vi "Test - Draw Teapot.vi"() -> ()   [LabVIEW 2022 SP3, in "Raster.lvlib"] (continued)
"Vertex 2"={"Position"={"x"=366.29727, "y"=442.02768, "z"=0.9899409}, "UV"={"u"=0.0, "v"=0.0}, "Colour"=12517256}, "Vertex 3"={"Position"={"x"=366.225, "y"=440.50778, "z"=0.990049}, "UV"={"u"=0.0, "v"=0.0}, "Colour"=12517256}, "Alpha"=0.0, "Alpha Blending Enabled"=FALSE, "Colour"=131841}, {"Vertex 1"={"Position"={"x"=433.7027, "y"=442.02768, "z"=0.9899409}, "UV"={"u"=0.0, "v"=0.0}, "Colour"=12517256}, "Vertex 2"={"Position"={"x"=437.2079, "y"=447.81754, "z"=0.98992956}, "UV"={"u"=0.0, "v"=0.0}, "Colour"=12517256}, "Vertex 3"={"Position"={"x"=437.24603, "y"=446.0728, "z"=0.990049}, "UV"={"u"=0.0, "v"=0.0}, "Colour"=12517256}, "Alpha"=0.0, "Alpha Blending Enabled"=FALSE, "Colour"=131841}, {"Vertex 1"={"Position"={"x"=379.34756, "y"=412.01456, "z"=0.98998296}, "UV"={"u"=0.0, "v"=0.0}, "Colour"=12517256}, "Vertex 2"={"Position"={"x"=382.73233, "y"=417.01996, "z"=0.98999375}, "UV"={"u"=0.0, "v"=0.0}, "Colour"=12517256}, "Vertex 3"={"Position"={"x"=383.29828, "y"=417.6338, "z"=0.989941}, "UV"={"u"=0.0, "v"=0.0}, "Colour"=12517256}, "Alpha"=0.0, "Alpha Blending Enabled"=FALSE, "Colour"=6588232}, {"Vertex 1"={"Position"={"x"=382.73233, "y"=417.01996, "z"=0.98999375}, "UV"={"u"=0.0, "v"=0.0}, "Colour"=12517256}, "Vertex 2"={"Position"={"x"=381.5074, "y"=422.85254, "z"=0.98998976}, "UV"={"u"=0.0, "v"=0.0}, "Colour"=12517256}, "Vertex 3"={"Position"={"x"=382.10587, "y"=423.5434, "z"=0.9899332}, "UV"={"u"=0.0, "v"=0.0}, "Colour"=12517256}, "Alpha"=0.0, "Alpha Blending Enabled"=FALSE, "Colour"=197634}, {"Vertex 1"={"Position"={"x"=498.9789, "y"=132.58115, "z"=0.990049}, "UV"={"u"=0.0, "v"=0.0}, "Colour"=12517256}, "Vertex 2"={"Position"={"x"=473.07867, "y"=131.5601, "z"=0.990049}, "UV"={"u"=0.0, "v"=0.0}, "Colour"=12517256}, "Vertex 3"={"Position"={"x"=473.84143, "y"=127.58133, "z"=0.9898128}, "UV"={"u"=0.0, "v"=0.0}, "Colour"=12517256}, "Alpha"=0.0, "Alpha Blending Enabled"=FALSE, "Colour"=131841}, {"Vertex 1"={"Position"={"x"=359.6493, "y"=130.9132, "z"=0.990049}, "UV"={"u"=0.0, "v"=0.0}, "Colour"=12517256}, "Vertex 2"={"Position"={"x"=326.92133, "y"=131.5601, "z"=0.990049}, "UV"={"u"=0.0, "v"=0.0}, "Colour"=12517256}, "Vertex 3"={"Position"={"x"=326.15854, "y"=127.58133, "z"=0.9898128}, "UV"={"u"=0.0, "v"=0.0}, "Colour"=12517256}, "Alpha"=0.0, "Alpha Blending Enabled"=FALSE, "Colour"=131841}, {"Vertex 1"={"Position"={"x"=362.81305, "y"=452.69107, "z"=0.9899296}, "UV"={"u"=0.0, "v"=0.0}, "Colour"=12517256}, "Vertex 2"={"Position"={"x"=362.7921, "y"=447.81754, "z"=0.98992956}, "UV"={"u"=0.0, "v"=0.0}, "Colour"=12517256}, "Vertex 3"={"Position"={"x"=362.754, "y"=446.0728, "z"=0.990049}, "UV"={"u"=0.0, "v"=0.0}, "Colour"=12517256}, "Alpha"=0.0, "Alpha Blending Enabled"=FALSE, "Colour"=724744}, {"Vertex 1"={"Position"={"x"=437.2079, "y"=447.81754, "z"=0.98992956}, "UV"={"u"=0.0, "v"=0.0}, "Colour"=12517256}, "Vertex 2"={"Position"={"x"=437.18695, "y"=452.69107, "z"=0.9899296}, "UV"={"u"=0.0, "v"=0.0}, "Colour"=12517256}, "Vertex 3"={"Position"={"x"=437.22525, "y"=450.8897, "z"=0.990049}, "UV"={"u"=0.0, "v"=0.0}, "Colour"=12517256}, "Alpha"=0.0, "Alpha Blending Enabled"=FALSE, "Colour"=724744}, {"Vertex 1"={"Position"={"x"=758.4817, "y"=387.64502, "z"=0.98992413}, "UV"={"u"=0.0, "v"=0.0}, "Colour"=12517256}, "Vertex 2"={"Position"={"x"=759.2145, "y"=388.6518, "z"=0.9899317}, "UV"={"u"=0.0, "v"=0.0}, "Colour"=12517256}, "Vertex 3"={"Position"={"x"=756.87177, "y"=387.67844, "z"=0.990049}, "UV"={"u"=0.0, "v"=0.0}, "Colour"=12517256}, "Alpha"=0.0, "Alpha Blending Enabled"=FALSE, "Colour"=131841}, {"Vertex 1"={"Position"={"x"=697.0016, "y"=386.77582, "z"=0.9899317}, "UV"={"u"=0.0, "v"=0.0}, "Colour"=12517256}, "Vertex 2"={"Position"={"x"=694.8843, "y"=386.1197, "z"=0.98992413}, "UV"={"u"=0.0, "v"=0.0}, "Colour"=12517256}, "Vertex 3"={"Position"={"x"=689.38416, "y"=385.0128, "z"=0.990049}, "UV"={"u"=0.0, "v"=0.0}, "Colour"=12517256}, "Alpha"=0.0, "Alpha Blending Enabled"=FALSE, "Colour"=9157219}, {"Vertex 1"={"Position"={"x"=422.71338, "y"=429.18945, "z"=0.98997617}, "UV"={"u"=0.0, "v"=0.0}, "Colour"=12517256}, "Vertex 2"={"Position"={"x"=418.4926, "y"=422.85254, "z"=0.98998976}, "UV"={"u"=0.0, "v"=0.0}, "Colour"=12517256}, "Vertex 3"={"Position"={"x"=417.89413, "y"=423.5434, "z"=0.9899332}, "UV"={"u"=0.0, "v"=0.0}, "Colour"=12517256}, "Alpha"=0.0, "Alpha Blending Enabled"=FALSE, "Colour"=131841}, {"Vertex 1"={"Position"={"x"=417.26767, "y"=417.01996, "z"=0.98999375}, "UV"={"u"=0.0, "v"=0.0}, "Colour"=12517256}, "Vertex 2"={"Position"={"x"=420.65244, "y"=412.01456, "z"=0.98998296}, "UV"={"u"=0.0, "v"=0.0}, "Colour"=12517256}, "Vertex 3"={"Position"={"x"=419.99554, "y"=412.71786, "z"=0.9899197}, "UV"={"u"=0.0, "v"=0.0}, "Colour"=12517256}, "Alpha"=0.0, "Alpha Blending Enabled"=FALSE, "Colour"=6653768}, {"Vertex 1"={"Position"={"x"=685.9131, "y"=304.15552, "z"=0.990049}, "UV"={"u"=0.0, "v"=0.0}, "Colour"=12517256}, "Vertex 2"={"Position"={"x"=679.2932, "y"=280.72607, "z"=0.990049}, "UV"={"u"=0.0, "v"=0.0}, "Colour"=12517256}, "Vertex 3"={"Position"={"x"=685.4334, "y"=281.3033, "z"=0.9897971}, "UV"={"u"=0.0, "v"=0.0}, "Colour"=12517256}, "Alpha"=0.0, "Alpha Blending Enabled"=FALSE, "Colour"=131841}, {"Vertex 1"={"Position"={"x"=641.6834, "y"=305.46494, "z"=0.990049}, "UV"={"u"=0.0, "v"=0.0}, "Colour"=12517256}, "Vertex 2"={"Position"={"x"=648.11633, "y"=317.74866, "z"=0.990049}, "UV"={"u"=0.0, "v"=0.0}, "Colour"=12517256}, "Vertex 3"={"Position"={"x"=655.26105, "y"=317.133, "z"=0.9897971}, "UV"={"u"=0.0, "v"=0.0}, "Colour"=12517256}, "Alpha"=0.0, "Alpha Blending Enabled"=FALSE, "Colour"=4941110}, {"Vertex 1"={"Position"={"x"=756.0784, "y"=386.048, "z"=0.9899179}, "UV"={"u"=0.0, "v"=0.0}, "Colour"=12517256}, "Vertex 2"={"Position"={"x"=758.4817, "y"=387.64502, "z"=0.98992413}, "UV"={"u"=0.0, "v"=0.0}, "Colour"=12517256}, "Vertex 3"={"Position"={"x"=755.92346, "y"=386.60867, "z"=0.990049}, "UV"={"u"=0.0, "v"=0.0}, "Colour"=12517256}, "Alpha"=0.0, "Alpha Blending Enabled"=FALSE, "Colour"=131841}, {"Vertex 1"={"Position"={"x"=694.8843, "y"=386.1197, "z"=0.98992413}, "UV"={"u"=0.0, "v"=0.0}, "Colour"=12517256}, "Vertex 2"={"Position"={"x"=692.3103, "y"=384.97452, "z"=0.9899179}, "UV"={"u"=0.0, "v"=0.0}, "Colour"=12517256}, "Vertex 3"={"Position"={"x"=686.6613, "y"=383.84372, "z"=0.990049}, "UV"={"u"=0.0, "v"=0.0}, "Colour"=12517256}, "Alpha"=0.0, "Alpha Blending Enabled"=FALSE, "Colour"=9025634}, {"Vertex 1"={"Position"={"x"=751.9063, "y"=383.8893, "z"=0.9899137}, "UV"={"u"=0.0, "v"=0.0}, "Colour"=12517256}, "Vertex 2"={"Position"={"x"=756.0784, "y"=386.048, "z"=0.9899179}, "UV"={"u"=0.0, "v"=0.0}, "Colour"=12517256}, "Vertex 3"={"Position"={"x"=753.3384, "y"=384.9661, "z"=0.990049}, "UV"={"u"=0.0, "v"=0.0}, "Colour"=12517256}, "Alpha"=0.0, "Alpha Blending Enabled"=FALSE, "Colour"=131841}, {"Vertex 1"={"Position"={"x"=692.3103, "y"=384.97452, "z"=0.9899179}, "UV"={"u"=0.0, "v"=0.0}, "Colour"=12517256}, "Vertex 2"={"Position"={"x"=689.3818, "y"=383.3356, "z"=0.9899137}, "UV"={"u"=0.0, "v"=0.0}, "Colour"=12517256}, "Vertex 3"={"Position"={"x"=683.68915, "y"=382.2069, "z"=0.990049}, "UV"={"u"=0.0, "v"=0.0}, "Colour"=12517256}, "Alpha"=0.0, "Alpha Blending Enabled"=FALSE, "Colour"=8828000}, {"Vertex 1"={"Position"={"x"=745.86945, "y"=381.19867, "z"=0.98991215}, "UV"={"u"=0.0, "v"=0.0}, "Colour"=12517256}, "Vertex 2"={"Position"={"x"=751.9063, "y"=383.8893, "z"=0.9899137}, "UV"={"u"=0.0, "v"=0.0}, "Colour"=12517256}, "Vertex 3"={"Position"={"x"=749.0386, "y"=382.78564, "z"=0.990049}, "UV"={"u"=0.0, "v"=0.0}, "Colour"=12517256}, "Alpha"=0.0, "Alpha Blending Enabled"=FALSE, "Colour"=131841}, {"Vertex 1"={"Position"={"x"=689.3818, "y"=383.3356, "z"=0.9899137}, "UV"={"u"=0.0, "v"=0.0}, "Colour"=12517256}, "Vertex 2"={"Position"={"x"=686.20184, "y"=381.19867, "z"=0.98991215}, "UV"={"u"=0.0, "v"=0.0}, "Colour"=12517256}, "Vertex 3"={"Position"={"x"=680.5922, "y"=380.10245, "z"=0.990049}, "UV"={"u"=0.0, "v"=0.0}, "Colour"=12517256}, "Alpha"=0.0, "Alpha Blending Enabled"=FALSE, "Colour"=8498525}, {"Vertex 1"={"Position"={"x"=381.5074, "y"=422.85254, "z"=0.98998976}, "UV"={"u"=0.0, "v"=0.0}, "Colour"=12517256}, "Vertex 2"={"Position"={"x"=377.28662, "y"=429.18945, "z"=0.98997617}, "UV"={"u"=0.0, "v"=0.0}, "Colour"=12517256}, "Vertex 3"={"Position"={"x"=377.9922, "y"=430.0834, "z"=0.98990643}, "UV"={"u"=0.0, "v"=0.0}, "Colour"=12517256}, "Alpha"=0.0, "Alpha Blending Enabled"=FALSE, "Colour"=131841}, {"Vertex 1"={"Position"={"x"=299.15308, "y"=393.3215, "z"=0.990049}, "UV"={"u"=0.0, "v"=0.0}, "Colour"=12517256}, "Vertex 2"={"Position"={"x"=314.2635, "y"=395.69092, "z"=0.990049}, "UV"={"u"=0.0, "v"=0.0}, "Colour"=12517256}, "Vertex 3"={"Position"={"x"=313.01276, "y"=398.35367, "z"=0.9897707}, "UV"={"u"=0.0, "v"=0.0}, "Colour"=12517256}, "Alpha"=0.0, "Alpha Blending Enabled"=FALSE, "Colour"=8828000}, {"Vertex 1"={"Position"={"x"=470.00256, "y"=398.0604, "z"=0.990049}, "UV"={"u"=0.0, "v"=0.0}, "Colour"=12517256}, "Vertex 2"={"Position"={"x"=485.7365, "y"=395.69092, "z"=0.990049}, "UV"={"u"=0.0, "v"=0.0}, "Colour"=12517256}, "Vertex 3"={"Position"={"x"=486.98724, "y"=398.35367, "z"=0.9897707}, "UV"={"u"=0.0, "v"=0.0}, "Colour"=12517256}, "Alpha"=0.0, "Alpha Blending Enabled"=FALSE, "Colour"=8828000}, {"Vertex 1"={"Position"={"x"=382.10587, "y"=423.5434, "z"=0.9899332}, "UV"={"u"=0.0, "v"=0.0}, "Colour"=12517256}, "Vertex 2"={"Position"={"x"=383.29828, "y"=417.6338, "z"=0.989941}, "UV"={"u"=0.0, "v"=0.0}, "Colour"=12517256}, "Vertex 3"={"Position"={"x"=382.73233, "y"=417.01996, "z"=0.98999375}, "UV"={"u"=0.0, "v"=0.0}, "Colour"=12517256}, "Alpha"=0.0, "Alpha Blending Enabled"=FALSE, "Colour"=197634}, {"Vertex 1"={"Position"={"x"=722.66376, "y"=367.07578, "z"=0.9899058}, "UV"={"u"=0.0, "v"=0.0}, "Colour"=12517256}, "Vertex 2"={"Position"={"x"=745.86945, "y"=381.19867, "z"=0.98991215}, "UV"={"u"=0.0, "v"=0.0}, "Colour"=12517256}, "Vertex 3"={"Position"={"x"=742.9461, "y"=380.10245, "z"=0.990049}, "UV"={"u"=0.0, "v"=0.0}, "Colour"=12517256}, "Alpha"=0.0, "Alpha Blending Enabled"=FALSE, "Colour"=131841}, {"Vertex 1"={"Position"={"x"=686.20184, "y"=381.19867, "z"=0.98991215}, "UV"={"u"=0.0, "v"=0.0}, "Colour"=12517256}, "Vertex 2"={"Position"={"x"=675.37756, "y"=370.58347, "z"=0.9899058}, "UV"={"u"=0.0, "v"=0.0}, "Colour"=12517256}, "Vertex 3"={"Position"={"x"=670.1064, "y"=369.6894, "z"=0.990049}, "UV"={"u"=0.0, "v"=0.0}, "Colour"=12517256}, "Alpha"=0.0, "Alpha Blending Enabled"=FALSE, "Colour"=7576146}, {"Vertex 1"={"Position"={"x"=416.7017, "y"=417.6338, "z"=0.989941}, "UV"={"u"=0.0, "v"=0.0}, "Colour"=12517256}, "Vertex 2"={"Position"={"x"=417.89413, "y"=423.5434, "z"=0.9899332}, "UV"={"u"=0.0, "v"=0.0}, "Colour"=12517256}, "Vertex 3"={"Position"={"x"=418.4926, "y"=422.85254, "z"=0.98998976}, "UV"={"u"=0.0, "v"=0.0}, "Colour"=12517256}, "Alpha"=0.0, "Alpha Blending Enabled"=FALSE, "Colour"=197634}, {"Vertex 1"={"Position"={"x"=679.2932, "y"=280.72607, "z"=0.990049}, "UV"={"u"=0.0, "v"=0.0}, "Colour"=12517256}, "Vertex 2"={"Position"={"x"=671.11444, "y"=257.76425, "z"=0.990049}, "UV"={"u"=0.0, "v"=0.0}, "Colour"=12517256}, "Vertex 3"={"Position"={"x"=678.03265, "y"=257.92834, "z"=0.98976254}, "UV"={"u"=0.0, "v"=0.0}, "Colour"=12517256}, "Alpha"=0.0, "Alpha Blending Enabled"=FALSE, "Colour"=131841}, {"Vertex 1"={"Position"={"x"=632.507, "y"=294.77127, "z"=0.990049}, "UV"={"u"=0.0, "v"=0.0}, "Colour"=12517256}, "Vertex 2"={"Position"={"x"=641.6834, "y"=305.46494, "z"=0.990049}, "UV"={"u"=0.0, "v"=0.0}, "Colour"=12517256}, "Vertex 3"={"Position"={"x"=649.45404, "y"=304.2476, "z"=0.98976254}, "UV"={"u"=0.0, "v"=0.0}, "Colour"=12517256}, "Alpha"=0.0, "Alpha Blending Enabled"=FALSE, "Colour"=6653768}, {"Vertex 1"={"Position"={"x"=371.0727, "y"=408.02982, "z"=0.9899565}, "UV"={"u"=0.0, "v"=0.0}, "Colour"=12517256}, "Vertex 2"={"Position"={"x"=379.34756, "y"=412.01456, "z"=0.98998296}, "UV"={"u"=0.0, "v"=0.0}, "Colour"=12517256}, "Vertex 3"={"Position"={"x"=380.00443, "y"=412.71786, "z"=0.9899197}, "UV"={"u"=0.0, "v"=0.0}, "Colour"=12517256}, "Alpha"=0.0, "Alpha Blending Enabled"=FALSE, "Colour"=8828000}, {"Vertex 1"={"Position"={"x"=419.99554, "y"=412.71786, "z"=0.9899197}, "UV"={"u"=0.0, "v"=0.0}, "Colour"=12517256}, "Vertex 2"={"Position"={"x"=416.7017, "y"=417.6338, "z"=0.989941}, "UV"={"u"=0.0, "v"=0.0}, "Colour"=12517256}, "Vertex 3"={"Position"={"x"=417.26767, "y"=417.01996, "z"=0.98999375}, "UV"={"u"=0.0, "v"=0.0}, "Colour"=12517256}, "Alpha"=0.0, "Alpha Blending Enabled"=FALSE, "Colour"=6588232}, {"Vertex 1"={"Position"={"x"=367.99426, "y"=456.267, "z"=0.98994625}, "UV"={"u"=0.0, "v"=0.0}, "Colour"=12517256}, "Vertex 2"={"Position"={"x"=379.90686, "y"=458.17007, "z"=0.9899845}, "UV"={"u"=0.0, "v"=0.0}, "Colour"=12517256}, "Vertex 3"={"Position"={"x"=380.54544, "y"=459.1382, "z"=0.9899229}, "UV"={"u"=0.0, "v"=0.0}, "Colour"=12517256}, "Alpha"=0.0, "Alpha Blending Enabled"=FALSE, "Colour"=9091427}, {"Vertex 1"={"Position"={"x"=383.29828, "y"=417.6338, "z"=0.989941}, "UV"={"u"=0.0, "v"=0.0}, "Colour"=12517256}, "Vertex 2"={"Position"={"x"=380.00443, "y"=412.71786, "z"=0.9899197}, "UV"={"u"=0.0, "v"=0.0}, "Colour"=12517256}, "Vertex 3"={"Position"={"x"=379.34756, "y"=412.01456, "z"=0.98998296}, "UV"={"u"=0.0, "v"=0.0}, "Colour"=12517256}, "Alpha"=0.0, "Alpha Blending Enabled"=FALSE, "Colour"=6588232}, {"Vertex 1"={"Position"={"x"=707.4174, "y"=348.9724, "z"=0.9898884}, "UV"={"u"=0.0, "v"=0.0}, "Colour"=12517256}, "Vertex 2"={"Position"={"x"=722.66376, "y"=367.07578, "z"=0.9899058}, "UV"={"u"=0.0, "v"=0.0}, "Colour"=12517256}, "Vertex 3"={"Position"={"x"=719.4906, "y"=366.02612, "z"=0.990049}, "UV"={"u"=0.0, "v"=0.0}, "Colour"=12517256}, "Alpha"=0.0, "Alpha Blending Enabled"=FALSE, "Colour"=131841}, {"Vertex 1"={"Position"={"x"=675.37756, "y"=370.58347, "z"=0.9899058}, "UV"={"u"=0.0, "v"=0.0}, "Colour"=12517256}, "Vertex 2"={"Position"={"x"=668.18396, "y"=358.2425, "z"=0.9898884}, "UV"={"u"=0.0, "v"=0.0}, "Colour"=12517256}, "Vertex 3"={"Position"={"x"=662.8006, "y"=357.59274, "z"=0.990049}, "UV"={"u"=0.0, "v"=0.0}, "Colour"=12517256}, "Alpha"=0.0, "Alpha Blending Enabled"=FALSE, "Colour"=5863232}, {"Vertex 1"={"Position"={"x"=359.34708, "y"=404.8941, "z"=0.98991895}, "UV"={"u"=0.0, "v"=0.0}, "Colour"=12517256}, "Vertex 2"={"Position"={"x"=345.11398, "y"=402.38348, "z"=0.9898734}, "UV"={"u"=0.0, "v"=0.0}, "Colour"=12517256}, "Vertex 3"={"Position"={"x"=345.35727, "y"=400.61688, "z"=0.990049}, "UV"={"u"=0.0, "v"=0.0}, "Colour"=12517256}, "Alpha"=0.0, "Alpha Blending Enabled"=FALSE, "Colour"=8827744}, {"Vertex 1"={"Position"={"x"=454.88602, "y"=402.38348, "z"=0.9898734}, "UV"={"u"=0.0, "v"=0.0}, "Colour"=12517256}, "Vertex 2"={"Position"={"x"=440.6529, "y"=404.8941, "z"=0.98991895}, "UV"={"u"=0.0, "v"=0.0}, "Colour"=12517256}, "Vertex 3"={"Position"={"x"=440.6547, "y"=403.54755, "z"=0.990049}, "UV"={"u"=0.0, "v"=0.0}, "Colour"=12517256}, "Alpha"=0.0, "Alpha Blending Enabled"=FALSE, "Colour"=8827744}, {"Vertex 1"={"Position"={"x"=428.32388, "y"=435.69714, "z"=0.9899581}, "UV"={"u"=0.0, "v"=0.0}, "Colour"=12517256}, "Vertex 2"={"Position"={"x"=422.71338, "y"=429.18945, "z"=0.98997617}, "UV"={"u"=0.0, "v"=0.0}, "Colour"=12517256}, "Vertex 3"={"Position"={"x"=422.0078, "y"=430.0834, "z"=0.98990643}, "UV"={"u"=0.0, "v"=0.0}, "Colour"=12517256}, "Alpha"=0.0, "Alpha Blending Enabled"=FALSE, "Colour"=131841}, {"Vertex 1"={"Position"={"x"=400.0, "y"=458.04477, "z"=0.990049}, "UV"={"u"=0.0, "v"=0.0}, "Colour"=12517256}, "Vertex 2"={"Position"={"x"=381.66364, "y"=460.0469, "z"=0.98986506}, "UV"={"u"=0.0, "v"=0.0}, "Colour"=12517256}, "Vertex 3"={"Position"={"x"=380.54544, "y"=459.1382, "z"=0.9899229}, "UV"={"u"=0.0, "v"=0.0}, "Colour"=12517256}, "Alpha"=0.0, "Alpha Blending Enabled"=FALSE, "Colour"=8959842}, {"Vertex 1"={"Position"={"x"=400.0, "y"=458.04477, "z"=0.990049}, "UV"={"u"=0.0, "v"=0.0}, "Colour"=12517256}, "Vertex 2"={"Position"={"x"=419.4546, "y"=459.1382, "z"=0.9899229}, "UV"={"u"=0.0, "v"=0.0}, "Colour"=12517256}, "Vertex 3"={"Position"={"x"=418.33633, "y"=460.0469, "z"=0.98986506}, "UV"={"u"=0.0, "v"=0.0}, "Colour"=12517256}, "Alpha"=0.0, "Alpha Blending Enabled"=FALSE, "Colour"=8959842}, {"Vertex 1"={"Position"={"x"=377.9922, "y"=430.0834, "z"=0.98990643}, "UV"={"u"=0.0, "v"=0.0}, "Colour"=12517256}, "Vertex 2"={"Position"={"x"=382.10587, "y"=423.5434, "z"=0.9899332}, "UV"={"u"=0.0, "v"=0.0}, "Colour"=12517256}, "Vertex 3"={"Position"={"x"=381.5074, "y"=422.85254, "z"=0.98998976}, "UV"={"u"=0.0, "v"=0.0}, "Colour"=12517256}, "Alpha"=0.0, "Alpha Blending Enabled"=FALSE, "Colour"=131841}, {"Vertex 1"={"Position"={"x"=671.11444, "y"=257.76425, "z"=0.990049}, "UV"={"u"=0.0, "v"=0.0}, "Colour"=12517256}, "Vertex 2"={"Position"={"x"=659.06976, "y"=236.3925, "z"=0.990049}, "UV"={"u"=0.0, "v"=0.0}, "Colour"=12517256}, "Vertex 3"={"Position"={"x"=666.5512, "y"=236.05386, "z"=0.9897306}, "UV"={"u"=0.0, "v"=0.0}, "Colour"=12517256}, "Alpha"=0.0, "Alpha Blending Enabled"=FALSE, "Colour"=131841}, {"Vertex 1"={"Position"={"x"=619.40234, "y"=286.3223, "z"=0.990049}, "UV"={"u"=0.0, "v"=0.0}, "Colour"=12517256}, "Vertex 2"={"Position"={"x"=632.507, "y"=294.77127, "z"=0.990049}, "UV"={"u"=0.0, "v"=0.0}, "Colour"=12517256}, "Vertex 3"={"Position"={"x"=640.6776, "y"=292.91815, "z"=0.9897306}, "UV"={"u"=0.0, "v"=0.0}, "Colour"=12517256}, "Alpha"=0.0, "Alpha Blending Enabled"=FALSE, "Colour"=8366683}, {"Vertex 1"={"Position"={"x"=518.84644, "y"=133.92955, "z"=0.990049}, "UV"={"u"=0.0, "v"=0.0}, "Colour"=12517256}, "Vertex 2"={"Position"={"x"=498.9789, "y"=132.58115, "z"=0.990049}, "UV"={"u"=0.0, "v"=0.0}, "Colour"=12517256}, "Vertex 3"={"Position"={"x"=500.85635, "y"=127.179695, "z"=0.98972636}, "UV"={"u"=0.0, "v"=0.0}, "Colour"=12517256}, "Alpha"=0.0, "Alpha Blending Enabled"=FALSE, "Colour"=131841}, {"Vertex 1"={"Position"={"x"=326.92133, "y"=131.5601, "z"=0.990049}, "UV"={"u"=0.0, "v"=0.0}, "Colour"=12517256}, "Vertex 2"={"Position"={"x"=301.0211, "y"=132.58115, "z"=0.990049}, "UV"={"u"=0.0, "v"=0.0}, "Colour"=12517256}, "Vertex 3"={"Position"={"x"=299.14365, "y"=127.179695, "z"=0.98972636}, "UV"={"u"=0.0, "v"=0.0}, "Colour"=12517256}, "Alpha"=0.0, "Alpha Blending Enabled"=FALSE, "Colour"=131841}, {"Vertex 1"={"Position"={"x"=285.66385, "y"=390.76498, "z"=0.990049}, "UV"={"u"=0.0, "v"=0.0}, "Colour"=12517256}, "Vertex 2"={"Position"={"x"=299.15308, "y"=393.3215, "z"=0.990049}, "UV"={"u"=0.0, "v"=0.0}, "Colour"=12517256}, "Vertex 3"={"Position"={"x"=297.17767, "y"=396.39102, "z"=0.98972005}, "UV"={"u"=0.0, "v"=0.0}, "Colour"=12517256}, "Alpha"=0.0, "Alpha Blending Enabled"=FALSE, "Colour"=8828000}, {"Vertex 1"={"Position"={"x"=485.7365, "y"=395.69092, "z"=0.990049}, "UV"={"u"=0.0, "v"=0.0}, "Colour"=12517256}, "Vertex 2"={"Position"={"x"=500.84695, "y"=393.3215, "z"=0.990049}, "UV"={"u"=0.0, "v"=0.0}, "Colour"=12517256}, "Vertex 3"={"Position"={"x"=502.8223, "y"=396.39102, "z"=0.98972005}, "UV"={"u"=0.0, "v"=0.0}, "Colour"=12517256}, "Alpha"=0.0, "Alpha Blending Enabled"=FALSE, "Colour"=8828000}, {"Vertex 1"={"Position"={"x"=176.70644, "y"=203.00851, "z"=0.9898844}, "UV"={"u"=0.0, "v"=0.0}, "Colour"=12517256}, "Vertex 2"={"Position"={"x"=198.99898, "y"=192.16704, "z"=0.9898844}, "UV"={"u"=0.0, "v"=0.0}, "Colour"=12517256}, "Vertex 3"={"Position"={"x"=202.54619, "y"=193.041, "z"=0.990049}, "UV"={"u"=0.0, "v"=0.0}, "Colour"=12517256}, "Alpha"=0.0, "Alpha Blending Enabled"=FALSE, "Colour"=131841}, {"Vertex 1"={"Position"={"x"=189.0271, "y"=222.08267, "z"=0.9898844}, "UV"={"u"=0.0, "v"=0.0}, "Colour"=12517256}, "Vertex 2"={"Position"={"x"=173.90924, "y"=229.9663, "z"=0.9898844}, "UV"={"u"=0.0, "v"=0.0}, "Colour"=12517256}, "Vertex 3"={"Position"={"x"=177.49036, "y"=231.8874, "z"=0.990049}, "UV"={"u"=0.0, "v"=0.0}, "Colour"=12517256}, "Alpha"=0.0, "Alpha Blending Enabled"=FALSE, "Colour"=8498525}, {"Vertex 1"={"Position"={"x"=156.89874, "y"=214.32089, "z"=0.9898844}, "UV"={"u"=0.0, "v"=0.0}, "Colour"=12517256}, "Vertex 2"={"Position"={"x"=176.70644, "y"=203.00851, "z"=0.9898844}, "UV"={"u"=0.0, "v"=0.0}, "Colour"=12517256}, "Vertex 3"={"Position"={"x"=180.40538, "y"=203.79315, "z"=0.990049}, "UV"={"u"=0.0, "v"=0.0}, "Colour"=12517256}, "Alpha"=0.0, "Alpha Blending Enabled"=FALSE, "Colour"=131841}, {"Vertex 1"={"Position"={"x"=173.90924, "y"=229.9663, "z"=0.9898844}, "UV"={"u"=0.0, "v"=0.0}, "Colour"=12517256}, "Vertex 2"={"Position"={"x"=160.64813, "y"=238.9713, "z"=0.9898844}, "UV"={"u"=0.0, "v"=0.0}, "Colour"=12517256}, "Vertex 3"={"Position"={"x"=164.63506, "y"=240.6793, "z"=0.990049}, "UV"={"u"=0.0, "v"=0.0}, "Colour"=12517256}, "Alpha"=0.0, "Alpha Blending Enabled"=FALSE, "Colour"=7971671}, {"Vertex 1"={"Position"={"x"=139.54333, "y"=226.07301, "z"=0.9898844}, "UV"={"u"=0.0, "v"=0.0}, "Colour"=12517256}, "Vertex 2"={"Position"={"x"=156.89874, "y"=214.32089, "z"=0.9898844}, "UV"={"u"=0.0, "v"=0.0}, "Colour"=12517256}, "Vertex 3"={"Position"={"x"=160.72755, "y"=214.98953, "z"=0.990049}, "UV"={"u"=0.0, "v"=0.0}, "Colour"=12517256}, "Alpha"=0.0, "Alpha Blending Enabled"=FALSE, "Colour"=131841}, {"Vertex 1"={"Position"={"x"=160.64813, "y"=238.9713, "z"=0.9898844}, "UV"={"u"=0.0, "v"=0.0}, "Colour"=12517256}, "Vertex 2"={"Position"={"x"=149.1812, "y"=248.82013, "z"=0.9898844}, "UV"={"u"=0.0, "v"=0.0}, "Colour"=12517256}, "Vertex 3"={"Position"={"x"=153.52568, "y"=250.31297, "z"=0.990049}, "UV"={"u"=0.0, "v"=0.0}, "Colour"=12517256}, "Alpha"=0.0, "Alpha Blending Enabled"=FALSE, "Colour"=7444305}, {"Vertex 1"={"Position"={"x"=124.60768, "y"=238.23384, "z"=0.9898844}, "UV"={"u"=0.0, "v"=0.0}, "Colour"=12517256}, "Vertex 2"={"Position"={"x"=139.54333, "y"=226.07301, "z"=0.9898844}, "UV"={"u"=0.0, "v"=0.0}, "Colour"=12517256}, "Vertex 3"={"Position"={"x"=143.48154, "y"=226.60681, "z"=0.990049}, "UV"={"u"=0.0, "v"=0.0}, "Colour"=12517256}, "Alpha"=0.0, "Alpha Blending Enabled"=FALSE, "Colour"=131841}, {"Vertex 1"={"Position"={"x"=149.1812, "y"=248.82013, "z"=0.9898844}, "UV"={"u"=0.0, "v"=0.0}, "Colour"=12517256}, "Vertex 2"={"Position"={"x"=139.44592, "y"=259.23462, "z"=0.9898844}, "UV"={"u"=0.0, "v"=0.0}, "Colour"=12517256}, "Vertex 3"={"Position"={"x"=144.09988, "y"=260.50784, "z"=0.990049}, "UV"={"u"=0.0, "v"=0.0}, "Colour"=12517256}, "Alpha"=0.0, "Alpha Blending Enabled"=FALSE, "Colour"=6785610}, {"Vertex 1"={"Position"={"x"=112.05928, "y"=250.77232, "z"=0.9898844}, "UV"={"u"=0.0, "v"=0.0}, "Colour"=12517256}, "Vertex 2"={"Position"={"x"=124.60768, "y"=238.23384, "z"=0.9898844}, "UV"={"u"=0.0, "v"=0.0}, "Colour"=12517256}, "Vertex 3"={"Position"={"x"=128.63612, "y"=238.62166, "z"=0.990049}, "UV"={"u"=0.0, "v"=0.0}, "Colour"=12517256}, "Alpha"=0.0, "Alpha Blending Enabled"=FALSE, "Colour"=131841}, {"Vertex 1"={"Position"={"x"=139.44592, "y"=259.23462, "z"=0.9898844}, "UV"={"u"=0.0, "v"=0.0}, "Colour"=12517256}, "Vertex 2"={"Position"={"x"=131.37982, "y"=269.93704, "z"=0.9898844}, "UV"={"u"=0.0, "v"=0.0}, "Colour"=12517256}, "Vertex 3"={"Position"={"x"=136.29527, "y"=270.98328, "z"=0.990049}, "UV"={"u"=0.0, "v"=0.0}, "Colour"=12517256}, "Alpha"=0.0, "Alpha Blending Enabled"=FALSE, "Colour"=6126915}, {"Vertex 1"={"Position"={"x"=101.86548, "y"=263.65726, "z"=0.9898844}, "UV"={"u"=0.0, "v"=0.0}, "Colour"=12517256}, "Vertex 2"={"Position"={"x"=112.05928, "y"=250.77232, "z"=0.9898844}, "UV"={"u"=0.0, "v"=0.0}, "Colour"=12517256}, "Vertex 3"={"Position"={"x"=116.16016, "y"=251.01059, "z"=0.990049}, "UV"={"u"=0.0, "v"=0.0}, "Colour"=12517256}, "Alpha"=0.0, "Alpha Blending Enabled"=FALSE, "Colour"=131841}, {"Vertex 1"={"Position"={"x"=131.37982, "y"=269.93704, "z"=0.9898844}, "UV"={"u"=0.0, "v"=0.0}, "Colour"=12517256}, "Vertex 2"={"Position"={"x"=124.920364, "y"=280.6494, "z"=0.9898844}, "UV"={"u"=0.0, "v"=0.0}, "Colour"=12517256}, "Vertex 3"={"Position"={"x"=130.04947, "y"=281.45874, "z"=0.990049}, "UV"={"u"=0.0, "v"=0.0}, "Colour"=12517256}, "Alpha"=0.0, "Alpha Blending Enabled"=FALSE, "Colour"=5402171}, {"Vertex 1"={"Position"={"x"=93.99359, "y"=276.8578, "z"=0.9898844}, "UV"={"u"=0.0, "v"=0.0}, "Colour"=12517256}, "Vertex 2"={"Position"={"x"=101.86548, "y"=263.65726, "z"=0.9898844}, "UV"={"u"=0.0, "v"=0.0}, "Colour"=12517256}, "Vertex 3"={"Position"={"x"=106.02248, "y"=263.75024, "z"=0.990049}, "UV"={"u"=0.0, "v"=0.0}, "Colour"=12517256}, "Alpha"=0.0, "Alpha Blending Enabled"=FALSE, "Colour"=131841}, {"Vertex 1"={"Position"={"x"=124.920364, "y"=280.6494, "z"=0.9898844}, "UV"={"u"=0.0, "v"=0.0}, "Colour"=12517256}, "Vertex 2"={"Position"={"x"=120.0052, "y"=291.09393, "z"=0.9898844}, "UV"={"u"=0.0, "v"=0.0}, "Colour"=12517256}, "Vertex 3"={"Position"={"x"=125.30017, "y"=291.65356, "z"=0.990049}, "UV"={"u"=0.0, "v"=0.0}, "Colour"=12517256}, "Alpha"=0.0, "Alpha Blending Enabled"=FALSE, "Colour"=4677427}, {"Vertex 1"={"Position"={"x"=88.41114, "y"=290.34256, "z"=0.9898844}, "UV"={"u"=0.0, "v"=0.0}, "Colour"=12517256}, "Vertex 2"={"Position"={"x"=93.99359, "y"=276.8578, "z"=0.9898844}, "UV"={"u"=0.0, "v"=0.0}, "Colour"=12517256}, "Vertex 3"={"Position"={"x"=98.19188, "y"=276.81717, "z"=0.990049}, "UV"={"u"=0.0, "v"=0.0}, "Colour"=12517256}, "Alpha"=0.0, "Alpha Blending Enabled"=FALSE, "Colour"=131841}, {"Vertex 1"={"Position"={"x"=120.0052, "y"=291.09393, "z"=0.9898844}, "UV"={"u"=0.0, "v"=0.0}, "Colour"=12517256}, "Vertex 2"={"Position"={"x"=116.571785, "y"=300.99258, "z"=0.9898844}, "UV"={"u"=0.0, "v"=0.0}, "Colour"=12517256}, "Vertex 3"={"Position"={"x"=121.985054, "y"=301.2872, "z"=0.990049}, "UV"={"u"=0.0, "v"=0.0}, "Colour"=12517256}, "Alpha"=0.0, "Alpha Blending Enabled"=FALSE, "Colour"=3820841}, {"Vertex 1"={"Position"={"x"=85.085556, "y"=304.08072, "z"=0.9898844}, "UV"={"u"=0.0, "v"=0.0}, "Colour"=12517256}, "Vertex 2"={"Position"={"x"=88.41114, "y"=290.34256, "z"=0.9898844}, "UV"={"u"=0.0, "v"=0.0}, "Colour"=12517256}, "Vertex 3"={"Position"={"x"=92.63716, "y"=290.18823, "z"=0.990049}, "UV"={"u"=0.0, "v"=0.0}, "Colour"=12517256}, "Alpha"=0.0, "Alpha Blending Enabled"=FALSE, "Colour"=131841}, {"Vertex 1"={"Position"={"x"=116.571785, "y"=300.99258, "z"=0.9898844}, "UV"={"u"=0.0, "v"=0.0}, "Colour"=12517256}, "Vertex 2"={"Position"={"x"=114.557556, "y"=310.0675, "z"=0.9898844}, "UV"={"u"=0.0, "v"=0.0}, "Colour"=12517256}, "Vertex 3"={"Position"={"x"=120.04168, "y"=310.0791, "z"=0.990049}, "UV"={"u"=0.0, "v"=0.0}, "Colour"=12517256}, "Alpha"=0.0, "Alpha Blending Enabled"=FALSE, "Colour"=2832927}, {"Vertex 1"={"Position"={"x"=83.98433, "y"=318.0409, "z"=0.9898844}, "UV"={"u"=0.0, "v"=0.0}, "Colour"=12517256}, "Vertex 2"={"Position"={"x"=85.085556, "y"=304.08072, "z"=0.9898844}, "UV"={"u"=0.0, "v"=0.0}, "Colour"=12517256}, "Vertex 3"={"Position"={"x"=89.32722, "y"=303.83978, "z"=0.990049}, "UV"={"u"=0.0, "v"=0.0}, "Colour"=12517256}, "Alpha"=0.0, "Alpha Blending Enabled"=FALSE, "Colour"=197634}, {"Vertex 1"={"Position"={"x"=114.557556, "y"=310.0675, "z"=0.9898844}, "UV"={"u"=0.0, "v"=0.0}, "Colour"=12517256}, "Vertex 2"={"Position"={"x"=113.89995, "y"=318.0409, "z"=0.9898844}, "UV"={"u"=0.0, "v"=0.0}, "Colour"=12517256}, "Vertex 3"={"Position"={"x"=119.407745, "y"=317.74866, "z"=0.990049}, "UV"={"u"=0.0, "v"=0.0}, "Colour"=12517256}, "Alpha"=0.0, "Alpha Blending Enabled"=FALSE, "Colour"=1646866}, {"Vertex 1"={"Position"={"x"=85.559654, "y"=330.7427, "z"=0.9898844}, "UV"={"u"=0.0, "v"=0.0}, "Colour"=12517256}, "Vertex 2"={"Position"={"x"=83.98433, "y"=318.0409, "z"=0.9898844}, "UV"={"u"=0.0, "v"=0.0}, "Colour"=12517256}, "Vertex 3"={"Position"={"x"=88.23085, "y"=317.74866, "z"=0.990049}, "UV"={"u"=0.0, "v"=0.0}, "Colour"=12517256}, "Alpha"=0.0, "Alpha Blending Enabled"=FALSE, "Colour"=1976598}, {"Vertex 1"={"Position"={"x"=113.89995, "y"=318.0409, "z"=0.9898844}, "UV"={"u"=0.0, "v"=0.0}, "Colour"=12517256}, "Vertex 2"={"Position"={"x"=115.16618, "y"=324.6623, "z"=0.9898844}, "UV"={"u"=0.0, "v"=0.0}, "Colour"=12517256}, "Vertex 3"={"Position"={"x"=120.644424, "y"=324.08536, "z"=0.990049}, "UV"={"u"=0.0, "v"=0.0}, "Colour"=12517256}, "Alpha"=0.0, "Alpha Blending Enabled"=FALSE, "Colour"=131841}, {"Vertex 1"={"Position"={"x"=90.28456, "y"=340.91348, "z"=0.9898844}, "UV"={"u"=0.0, "v"=0.0}, "Colour"=12517256}, "Vertex 2"={"Position"={"x"=85.559654, "y"=330.7427, "z"=0.9898844}, "UV"={"u"=0.0, "v"=0.0}, "Colour"=12517256}, "Vertex 3"={"Position"={"x"=89.7897, "y"=330.4221, "z"=0.990049}, "UV"={"u"=0.0, "v"=0.0}, "Colour"=12517256}, "Alpha"=0.0, "Alpha Blending Enabled"=FALSE, "Colour"=4611634}, {"Vertex 1"={"Position"={"x"=115.16618, "y"=324.6623, "z"=0.9898844}, "UV"={"u"=0.0, "v"=0.0}, "Colour"=12517256}, "Vertex 2"={"Position"={"x"=118.92371, "y"=329.9643, "z"=0.9898844}, "UV"={"u"=0.0, "v"=0.0}, "Colour"=12517256}, "Vertex 3"={"Position"={"x"=124.31293, "y"=329.15936, "z"=0.990049}, "UV"={"u"=0.0, "v"=0.0}, "Colour"=12517256}, "Alpha"=0.0, "Alpha Blending Enabled"=FALSE, "Colour"=131841}, {"Vertex 1"={"Position"={"x"=98.157074, "y"=348.83447, "z"=0.9898844}, "UV"={"u"=0.0, "v"=0.0}, "Colour"=12517256}, "Vertex 2"={"Position"={"x"=90.28456, "y"=340.91348, "z"=0.9898844}, "UV"={"u"=0.0, "v"=0.0}, "Colour"=12517256}, "Vertex 3"={"Position"={"x"=94.46621, "y"=340.57016, "z"=0.990049}, "UV"={"u"=0.0, "v"=0.0}, "Colour"=12517256}, "Alpha"=0.0, "Alpha Blending Enabled"=FALSE, "Colour"=7049293}, {"Vertex 1"={"Position"={"x"=118.92371, "y"=329.9643, "z"=0.9898844}, "UV"={"u"=0.0, "v"=0.0}, "Colour"=12517256}, "Vertex 2"={"Position"={"x"=125.11115, "y"=334.09354, "z"=0.9898844}, "UV"={"u"=0.0, "v"=0.0}, "Colour"=12517256}, "Vertex 3"={"Position"={"x"=130.35083, "y"=333.11105, "z"=0.990049}, "UV"={"u"=0.0, "v"=0.0}, "Colour"=12517256}, "Alpha"=0.0, "Alpha Blending Enabled"=FALSE, "Colour"=131841}, {"Vertex 1"={"Position"={"x"=109.17566, "y"=354.78696, "z"=0.9898844}, "UV"={"u"=0.0, "v"=0.0}, "Colour"=12517256}, "Vertex 2"={"Position"={"x"=98.157074, "y"=348.83447, "z"=0.9898844}, "UV"={"u"=0.0, "v"=0.0}, "Colour"=12517256}, "Vertex 3"={"Position"={"x"=102.260445, "y"=348.47348, "z"=0.990049}, "UV"={"u"=0.0, "v"=0.0}, "Colour"=12517256}, "Alpha"=0.0, "Alpha Blending Enabled"=FALSE, "Colour"=8564317}, {"Vertex 1"={"Position"={"x"=125.11115, "y"=334.09354, "z"=0.9898844}, "UV"={"u"=0.0, "v"=0.0}, "Colour"=12517256}, "Vertex 2"={"Position"={"x"=133.66658, "y"=337.1965, "z"=0.9898844}, "UV"={"u"=0.0, "v"=0.0}, "Colour"=12517256}, "Vertex 3"={"Position"={"x"=138.69586, "y"=336.0807, "z"=0.990049}, "UV"={"u"=0.0, "v"=0.0}, "Colour"=12517256}, "Alpha"=0.0, "Alpha Blending Enabled"=FALSE, "Colour"=131841}, {"Vertex 1"={"Position"={"x"=123.33839, "y"=359.05215, "z"=0.9898844}, "UV"={"u"=0.0, "v"=0.0}, "Colour"=12517256}, "Vertex 2"={"Position"={"x"=109.17566, "y"=354.78696, "z"=0.9898844}, "UV"={"u"=0.0, "v"=0.0}, "Colour"=12517256}, "Vertex 3"={"Position"={"x"=113.172386, "y"=354.4127, "z"=0.990049}, "UV"={"u"=0.0, "v"=0.0}, "Colour"=12517256}, "Alpha"=0.0, "Alpha Blending Enabled"=FALSE, "Colour"=9157476}, {"Vertex 1"={"Position"={"x"=133.66658, "y"=337.1965, "z"=0.9898844}, "UV"={"u"=0.0, "v"=0.0}, "Colour"=12517256}, "Vertex 2"={"Position"={"x"=144.52863, "y"=339.41995, "z"=0.9898844}, "UV"={"u"=0.0, "v"=0.0}, "Colour"=12517256}, "Vertex 3"={"Position"={"x"=149.28564, "y"=338.2085, "z"=0.990049}, "UV"={"u"=0.0, "v"=0.0}, "Colour"=12517256}, "Alpha"=0.0, "Alpha Blending Enabled"=FALSE, "Colour"=131841}, {"Vertex 1"={"Position"={"x"=140.6435, "y"=361.91113, "z"=0.9898844}, "UV"={"u"=0.0, "v"=0.0}, "Colour"=12517256}, "Vertex 2"={"Position"={"x"=123.33839, "y"=359.05215, "z"=0.9898844}, "UV"={"u"=0.0, "v"=0.0}, "Colour"=12517256}, "Vertex 3"={"Position"={"x"=127.20199, "y"=358.6683, "z"=0.990049}, "UV"={"u"=0.0, "v"=0.0}, "Colour"=12517256}, "Alpha"=0.0, "Alpha Blending Enabled"=FALSE, "Colour"=9420902}, {"Vertex 1"={"Position"={"x"=144.52863, "y"=339.41995, "z"=0.9898844}, "UV"={"u"=0.0, "v"=0.0}, "Colour"=12517256}, "Vertex 2"={"Position"={"x"=157.63564, "y"=340.9104, "z"=0.9898844}, "UV"={"u"=0.0, "v"=0.0}, "Colour"=12517256}, "Vertex 3"={"Position"={"x"=162.05779, "y"=339.6349, "z"=0.990049}, "UV"={"u"=0.0, "v"=0.0}, "Colour"=12517256}, "Alpha"=0.0, "Alpha Blending Enabled"=FALSE, "Colour"=131841}, {"Vertex 1"={"Position"={"x"=161.08936, "y"=363.6454, "z"=0.9898844}, "UV"={"u"=0.0, "v"=0.0}, "Colour"=12517256}, "Vertex 2"={"Position"={"x"=140.6435, "y"=361.91113, "z"=0.9898844}, "UV"={"u"=0.0, "v"=0.0}, "Colour"=12517256}, "Vertex 3"={"Position"={"x"=144.34929, "y"=361.5211, "z"=0.990049}, "UV"={"u"=0.0, "v"=0.0}, "Colour"=12517256}, "Alpha"=0.0, "Alpha Blending Enabled"=FALSE, "Colour"=9486695}, {"Vertex 1"={"Position"={"x"=157.63564, "y"=340.9104, "z"=0.9898844}, "UV"={"u"=0.0, "v"=0.0}, "Colour"=12517256}, "Vertex 2"={"Position"={"x"=172.92587, "y"=341.81445, "z"=0.9898844}, "UV"={"u"=0.0, "v"=0.0}, "Colour"=12517256}, "Vertex 3"={"Position"={"x"=176.94994, "y"=340.5, "z"=0.990049}, "UV"={"u"=0.0, "v"=0.0}, "Colour"=12517256}, "Alpha"=0.0, "Alpha Blending Enabled"=FALSE, "Colour"=131841}, {"Vertex 1"={"Position"={"x"=184.6739, "y"=364.53586, "z"=0.9898844}, "UV"={"u"=0.0, "v"=0.0}, "Colour"=12517256}, "Vertex 2"={"Position"={"x"=161.08936, "y"=363.6454, "z"=0.9898844}, "UV"={"u"=0.0, "v"=0.0}, "Colour"=12517256}, "Vertex 3"={"Position"={"x"=164.61427, "y"=363.25134, "z"=0.990049}, "UV"={"u"=0.0, "v"=0.0}, "Colour"=12517256}, "Alpha"=0.0, "Alpha Blending Enabled"=FALSE, "Colour"=9486951}, {"Vertex 1"={"Position"={"x"=172.92587, "y"=341.81445, "z"=0.9898844}, "UV"={"u"=0.0, "v"=0.0}, "Colour"=12517256}, "Vertex 2"={"Position"={"x"=190.33804, "y"=342.2787, "z"=0.9898844}, "UV"={"u"=0.0, "v"=0.0}, "Colour"=12517256}, "Vertex 3"={"Position"={"x"=193.8998, "y"=340.9443, "z"=0.990049}, "UV"={"u"=0.0, "v"=0.0}, "Colour"=12517256}, "Alpha"=0.0, "Alpha Blending Enabled"=FALSE, "Colour"=131841}, {"Vertex 1"={"Position"={"x"=211.39569, "y"=364.86395, "z"=0.9898844}, "UV"={"u"=0.0, "v"=0.0}, "Colour"=12517256}, "Vertex 
